vi "transmit.vi"(8 "error in (no error)":errorcluster, 11 "Publisher in":refnum<class "Publisher.lvclass">) -> (0 "error out":errorcluster, 3 "Publisher out":refnum<class "Publisher.lvclass">)   [LabVIEW 2016, in "Publisher.lvclass"]
uses:
  Publisher.lvclass
  Publisher.lvclass/Publisher.ctl
  Communicator/M1M3SAL/M1M3SAL.lvclass/M1M3SAL.ctl
  Communicator/M1M3SAL/write.vi
  Communicator/M1M3SAL/M1M3SAL.lvclass
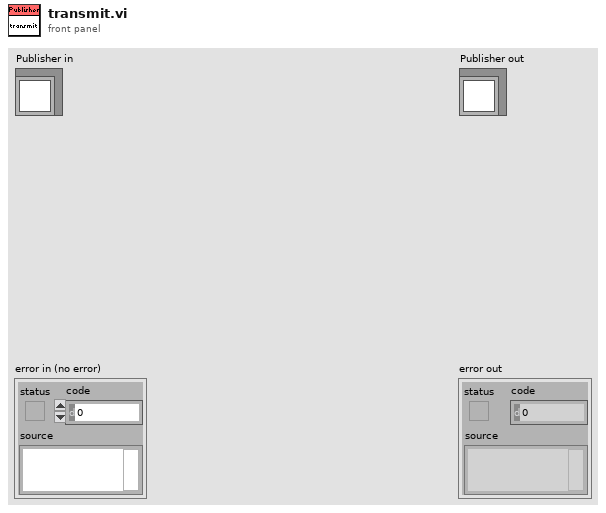
[diagram p1: front panel]
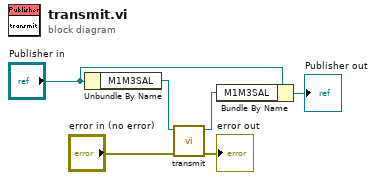
[diagram p0: block diagram]
diagram:
  n1 = Unbundle By Name("Publisher in") -> ("M1M3SAL"=w5:refnum<class "M1M3SAL.lvclass">)
  n2 = call "transmit.vi"("error in (no error)"="error in (no error)", "M1M3SAL in"=w5) -> ("error out"=→"error out":errorcluster, "M1M3SAL out"=w4:refnum<class "M1M3SAL.lvclass">)  [unwired: 8 in]
  n3 = Bundle By Name(cluster="Publisher in", "M1M3SAL"=w4) -> (→"Publisher out":refnum<class "Publisher.lvclass">)
